vi "Read Std Status Reg.vi"(8 "error in":errorcluster, 11 "SR 3XX HVPS in":refnum<class "SR 3XX HVPS.lvclass">) -> (0 "error out":errorcluster, 2 "StdEvntStatus":T1, 3 "SR 3XX HVPS out":refnum<class "SR 3XX HVPS.lvclass">)   [LabVIEW 2013, in "SR 3XX HVPS.lvclass"]
doc: "This status byte is defined by IEEE-488.2 (1987) and is used primarily to report errors in commands received over the communications interfaces. The bits in this register stay set once set and are cleared by reading them or by the *CLS command. If a bit in the standard status register is set and the corresponding bit in the\nstandard status enable register is set, then the ESB bit in the serial poll register is set.\n\nThe following error messages will appear on the middle display if an error occurs due to a command sent over GPIB:\n\n<B>Err6</B> Syntax Error over GPIB.\nThe command had an error in syntax or was unrecognizable. A syntax error could be a misspelling of a command or forgetting to include a '-' when setting a negative value for the voltage or voltage limit. This error is the same as Command Error, bit 5 of the Standard Event Status Byte.\n<B>Err7</B> Illegal Parameter entered over GPIB.\nA parameter was set out of range, or a command could not be completed because of an overload. This error is the same as Execution Err, bit 4 of the Standard Event Status Byte.\n<B>Err8</B> GPIB Output Queue full.\nThe output queue overflowed and was cleared. This could be due to querying the unit repeatedly and not reading out all of the characters, or a problem at the recieving unit. This error is the same as Query Error, bit 2 of the Standard Event Status Byte."
uses:
  SR 3XX HVPS.lvclass
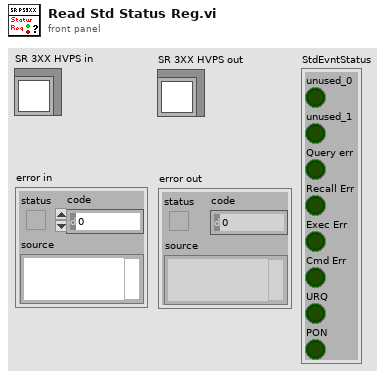
[diagram p1: front panel]
types:
  T1 = cluster{"unused_0":bool, "unused_1":bool, "Query err":bool, "Recall Err":bool, "Exec Err":bool, "Cmd Err":bool, "URQ":bool, "PON":bool}
  T2 = cluster{"Boolean array[0]":bool, "Boolean array[1]":bool, "Boolean array[2]":bool, "Boolean array[3]":bool, "Boolean array[4]":bool, "Boolean array[5]":bool, "Boolean array[6]":bool, "Boolean array[7]":bool}
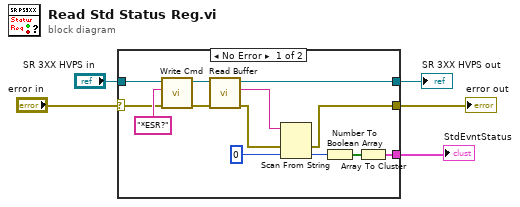
[diagram p0: block diagram]
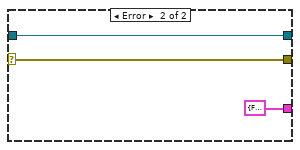
[diagram p2: hidden frame]
diagram:
  n1 = case shown="No Error" "error in" {
    selector: "error in" -> [w16 w21]
    tunnel: [w8 w21] -> w4
    tunnel: [w13 w20] -> w2
    tunnel: "SR 3XX HVPS in" -> [w18 w20]
    tunnel: [w6 T2 {"Boolean array[0]"=FALSE, "Boolean array[1]"=FALSE, "Boolean array[2]"=FALSE, "Boolean array[3]"=FALSE, "Boolean array[4]"=FALSE, "Boolean array[5]"=FALSE, "Boolean array[6]"=FALSE, "Boolean array[7]"=FALSE} ("Boolean array")] -> w1
    frame No Error {
      n2 = call "Write Cmd.vi"("error in"=w16, "Cmd"="*ESR?", "SR 3XX HVPS in"=w18) -> ("error out"=w14:errorcluster, "SR 3XX HVPS out"=w15:refnum<class "SR 3XX HVPS.lvclass">)  [unwired: 7 in]
      n3 = call "Read Buffer.vi"("error in"=w14, "SR 3XX HVPS in"=w15) -> ("error out"=w9:errorcluster, "ReadData"=w12:string, "SR 3XX HVPS out"=w13:refnum<class "SR 3XX HVPS.lvclass">)  [unwired: 7 in]
      n4 = Scan From String(input string=w12, error in=w9, default 1=u8 0 ("default value 1")) -> (error out=w8:errorcluster, output 1=w10:u8)  [unwired: 2 in, 2 out]
      n5 = Number To Boolean Array(number=w10) -> (Boolean array=w7:bool[])
      n6 = Array To Cluster(array=w7) -> (cluster=w6:T2)
    }
    frame Error {
    }
  }
  "error out" <- w4
  "SR 3XX HVPS out" <- w2
  "StdEvntStatus" <- w1
